vi "SS Write Read Test.vi"(10 "Numeric  Array to Write":dbl[][](array[numeric])=[[2.0, 5.0, 7.0], [1.0, 3.0, 9.0], [4.0, 5.0, 7.0]] format="%.2f") -> ()   [LabVIEW 2017]
panel:
  in  "Transpose Read":bool
  in  "Transpose Write":bool
  in  "Header String to Write":string="File Header String"
  out "Header String Read":string
  out "Numeric Array Read":dbl[][](array[numeric]) format="%.2f"
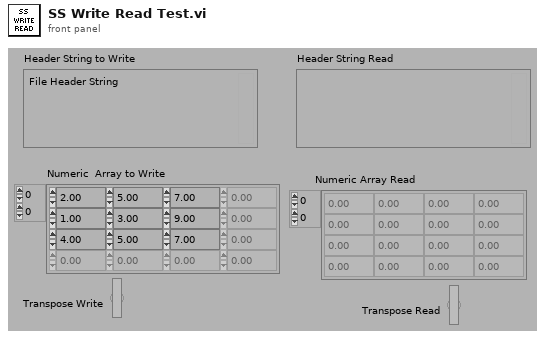
[diagram p1: front panel]
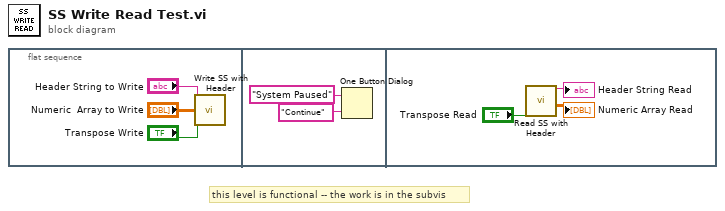
[diagram p0: block diagram]
diagram:
  # "this level is functional -- the work is in the subvis"
  n1 = flat-sequence {
    frame #0 {
      n2 = call "Write SS with Header.vi"("Header String"="Header String to Write", "Data to Write"="Numeric  Array to Write", "Transpose Data?"="Transpose Write") -> ()  [unwired: 13 in]
    }
    frame #1 {
      n3 = One Button Dialog(message="System Paused", button name ("OK")="Continue") -> ()  [unwired: 1 out]
    }
    frame #2 {
      n4 = call "Read SS with Header.vi"("Transpose Data Array"="Transpose Read") -> ("Header String"=→"Header String Read":string, "Data Read"=→"Numeric Array Read":dbl[][])  [unwired: 12 in, 1 out]
    }
  }
